vi "HRTF-Apply Window.vi"(0 "Array in":cdb[](array[numeric]), 7 "Window":T1, 9 "Fs (Hz)":dbl) -> (4 "Array out":cdb[](array[numeric]))   [LabVIEW 2015]
uses:
  Typedefs/HRTF-Window.ctl
  Typedefs/HRTF-Window Type.ctl
  <vilib>/Analysis/2dsp.llb/Inverse Real FFT.vi
  <vilib>/Analysis/4window.llb/Hanning Window (DBL).vi
  <vilib>/Analysis/2dsp.llb/Real FFT.vi
  <vilib>/Analysis/baseanly.llb/Mean.vi
  <vilib>/Analysis/baseanly.llb/Mean (DBL).vi
  <vilib>/Analysis/4window.llb/AllCosWindow (DBL).vi
  <vilib>/Analysis/NI_AALPro.lvlib
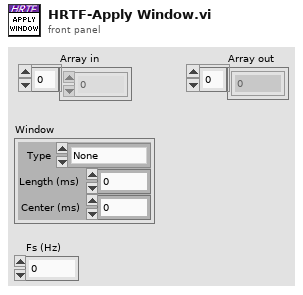
[diagram p1: front panel]
types:
  T1 = typedef "HRTF-Window.ctl" = cluster{"Type":T2, "Length (ms)":dbl, "Center (ms)":dbl}
  T2 = typedef "HRTF-Window Type.ctl" = enum16{"None", "Rectangle", "Hanning"}
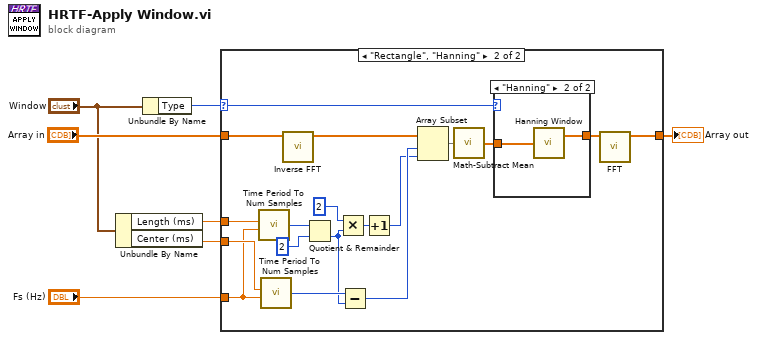
[diagram p0: block diagram]
diagram:
  n1 = Unbundle By Name("Window") -> ("Length (ms)"=w5:dbl, "Center (ms)"=w4:dbl)
  n2 = Unbundle By Name("Window") -> ("Type"=w2:T2)
  n3 = case shown="\"Rectangle\", \"Hanning\"" w2 {
    selector: w2 -> [_ w9]
    tunnel: "Array in" -> [w8 w20]
    tunnel: [w8 w19] -> w6
    tunnel: w5 -> [_ w26]
    tunnel: w4 -> [_ w25]
    tunnel: "Fs (Hz)" -> [_ w24]
    frame "None", Default {
    }
    frame "Rectangle", "Hanning" {
      n4 = call "Time Period To Num Samples.vi"("Duration (ms)"=w26, "Sampling rate (Hz)"=w24) -> ("Samples"=w22:i32)  [unwired: 5 in]
      n5 = call "Time Period To Num Samples.vi"("Duration (ms)"=w25, "Sampling rate (Hz)"=w24) -> ("Samples"=w21:i32)  [unwired: 5 in]
      n6 = call-poly <vilib>:"Inverse FFT.vi"("FFT {X}"=w20) -> ("X"=w10:dbl[])  [unwired: 9 in, 1 out]
      n7 = Quotient & Remainder(x=w22, y=2) -> (floor(x/y)=w17:i32)  [unwired: 1 out]
      n8 = Multiply(x=2, y=w17) -> (x*y=w15:i32)
      n9 = Subtract(x=w21, y=w17) -> (x-y=w14:i32)
      n10 = Increment(x=w15) -> (x+1=w11:i32)
      n11 = Array Subset(array=w10, index=w14, length=w11) -> (w13:dbl[])
      n12 = call "Math-Subtract Mean.vi"("Y"=w13) -> ("Y - mean(Y)"=w12:dbl[])  [unwired: 4 in]
      n13 = case shown="\"Hanning\"" w9 {
        tunnel: [w27 w29] -> w18
        tunnel: w12 -> [w27 w28]
        frame "None", Default {
        }
        frame "Hanning" {
          n14 = call-poly <vilib>:"Hanning Window.vi"("X"=w28) -> ("Windowed X"=w29:dbl[])  [unwired: 1 out]
        }
      }
      n15 = call-poly <vilib>:"FFT.vi"("X"=w18) -> ("FFT {X}"=w19:cdb[])  [unwired: 9 in, 1 out]
    }
  }
  "Array out" <- w6
